vi "Connect.vi"(8 "error in":errorcluster, 11 "6032A in":refnum<class "6032A.lvclass">) -> (0 "error out":errorcluster, 3 "6032A out":refnum<class "6032A.lvclass">)   [LabVIEW 2019, in "6032A.lvlib" / "6032A.lvclass"]
doc: "This disconnect routine is a must override from the Instrument Class\nChildren Classes are responsible for handling the override, but the parent class is an intermediary and must contain the override functions to maintain the rules for the method."
uses:
  Library/6032A.lvclass
  C:/Users/Public/Documents/Development/builds/Instruments/Instruments.lvlibp/Library/Instruments.lvclass
  Library/6032A.lvclass/6032A.ctl
  builds/Instruments/Instruments.lvlibp/Accessors/Read Resource.vi
  builds/Instruments/PowerSupply.lvlibp/Library/PowerSupply.lvclass
  <instrlib>/Agilent 6XXX Series/Agilent 6XXX Series.lvlib
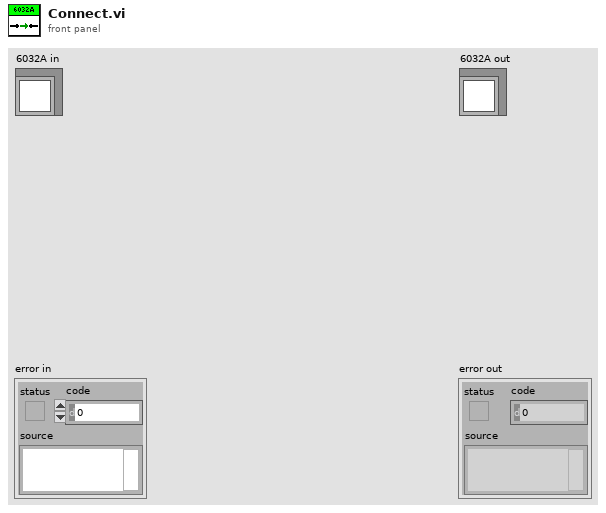
[diagram p1: front panel]
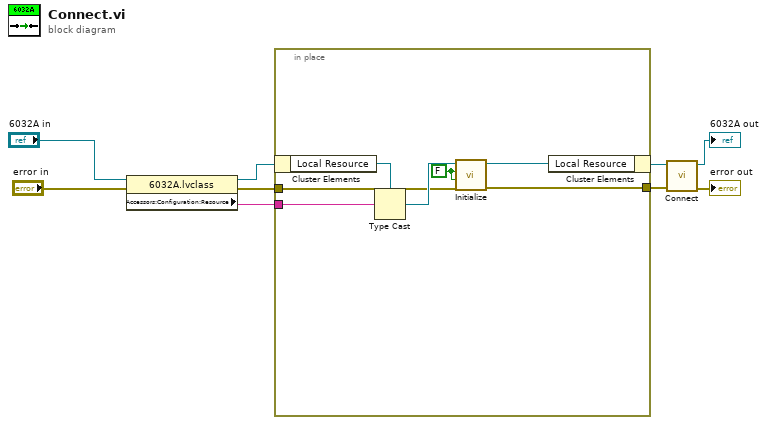
[diagram p0: block diagram]
diagram:
  n1 = property class="6032A.lvclass"(reference="6032A in", error in="error in") -> (reference out=w5:refnum<class "6032A.lvclass">, error out=w2:errorcluster, "Accessors:Configuration:Resource"=w3:string)
  n2 = in-place {
    in-place-border: w3 -> [w14]
    in-place-border: w2 -> [w12]
    in-place-border: [w11] -> w1
    w10 = FALSE ("ID Query (T: Check)")
    n3 = in-place-cluster #1(w5) -> ("Local Resource"=w15:refnum<visa-resource-name>)
    n4 = Type Cast(type=w15, x=w14) -> (*(type *) &x=w13:refnum<visa-resource-name>)
    n5 = call <instrlib>:"Initialize.vi"("error in (no error)"=w12, "Reset (T: Reset)"=w10, "ID Query (T: Check)"=w10, "VISA resource name"=w13) -> ("error out"=w11:errorcluster, "VISA resource name out"=w16:refnum<visa-resource-name>)  [unwired: 6 in]
    n6 = in-place-cluster #1("Local Resource"=w16) -> (w4:refnum<class "6032A.lvclass">)
  }
  n7 = call-parent "Connect.vi"("error in"=w1, "PowerSupply in"=w4) -> ("error out"=→"error out":errorcluster, "PowerSupply out"=→"6032A out":refnum<class "6032A.lvclass">)  [unwired: 8 in]
